vi "Unlock ECU Security.vi"(6 "Diagnostic Protocol":T2, 8 "error in (no error)":errorcluster, 10 "Security":T1={"Source DLL Path"=path "", "Security Level"=1, "Target DLL Path"=path ""}, 11 "diag ref in":T3) -> (0 "error out":errorcluster, 1 "success?":bool, 3 "diag ref out":T3)   [LabVIEW 2015, in "Diagnostics Addon Engine.lvlib"]
uses:
  Diagnostics Addon Engine.lvlib
  <vilib>/Automotive Diagnostic Command Set/Diagnostic Transport.llb/Diag Reference.ctl
  <vilib>/Automotive Diagnostic Command Set/Diagnostic Transport.llb/Transport Protocol Selector.ctl
  <vilib>/Automotive Diagnostic Command Set/Diagnostic Transport.llb/Diag CAN Frame Log.ctl
  Shared/Diagnostic Protocols.ctl
  Shared/Security.ctl
  GMLAN/_SubVIs/SecurityAccess_sendKey.vi
  GMLAN/_SubVIs/SecurityAccess_requestSeed.vi
  <vilib>/Automotive Diagnostic Command Set/Diagnostic Transport.llb/Apply Success Failure Error.vi
  <vilib>/Automotive Diagnostic Command Set/Diagnostic Transport.llb/Diagnostic Service.vi
  GMLAN/GMLAN.lvlib
  <vilib>/addons/Automotive Diagnostic Command Set/NI_Automotive Diagnostic Command Set.lvlib
  Shared/Diagnostics Addon Shared.lvlib
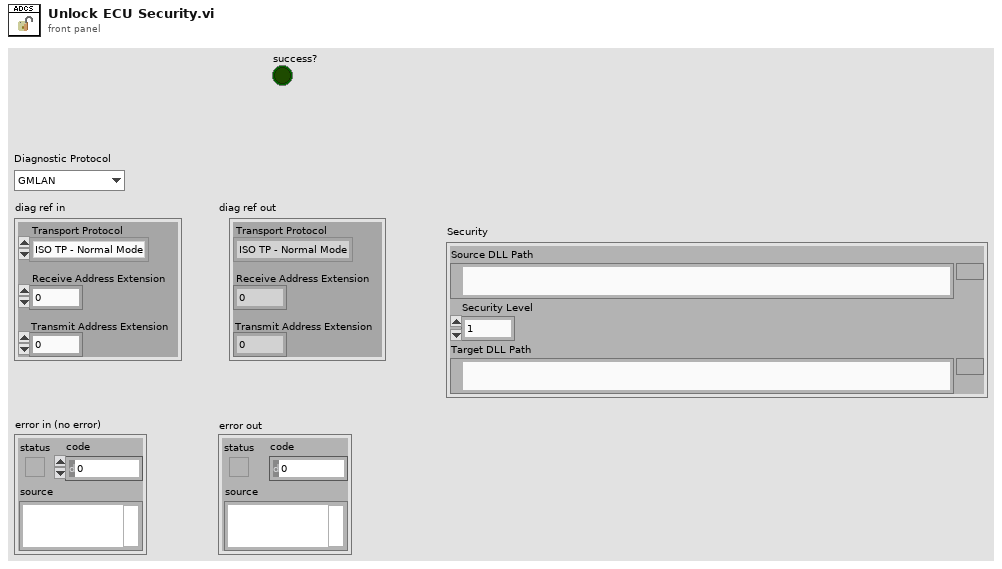
[diagram p1: front panel]
types:
  T1 = typedef "Diagnostics Addon Shared.lvlib/Security.ctl" = cluster{"Source DLL Path":path, "Security Level":u8, "Target DLL Path":path}
  T2 = typedef "Diagnostics Addon Shared.lvlib/Diagnostic Protocols.ctl" = enum16{"GMLAN", "KWP-2000", "UDS"}
  T3 = typedef "NI_Automotive Diagnostic Command Set.lvlib/Diag Reference.ctl" = cluster{"Diag CAN Handle":u32, "Transport Protocol":T4, "Receive Address Extension":u8, "Transmit Address Extension":u8, "Receive CAN Id":u32, "Transmit CAN Id":u32, "Diag CAN Queue":refnum<queue>, "Log Frames ?":bool, "My TP Address":u8, "Other TP Address":u8, "T1":u16, "T2":u16, "T3":u16, "T4":u16, "Tx SN":u8, "Block Size":u8, "Rx SN":u8, "VW TP Initialized?":bool, "Tx block no":u8, "baud rate":u32, "Interface":string, "Channel Diag CAN Handle":u32, "UDP Connection ID":refnum<k16>, "TCP Connection ID":refnum<k5>, "Target IP Addr":u32, "Source Address":u16, "Target Address":u16, "Send Header NACK?":bool, "DLL Handle":u32, "NAD":u8, "Time Stamp read first":dbl, "Time Stamp read last":dbl, "Time Stamp write first":dbl, "Time Stamp write last":dbl, "Time Stamp write":dbl, "Time Stamp read":dbl}
  T4 = typedef "NI_Automotive Diagnostic Command Set.lvlib/Transport Protocol Selector.ctl" = enum16{"ISO TP - Normal Mode", "ISO TP - Mixed Mode", "VW TP 2.0", "Diagnostics on IP", "ISO TP LIN"}
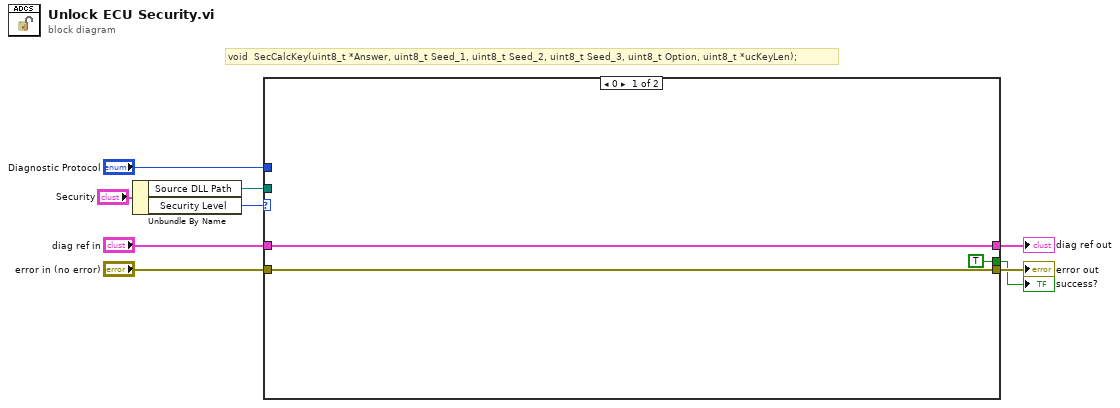
[diagram p0: block diagram]
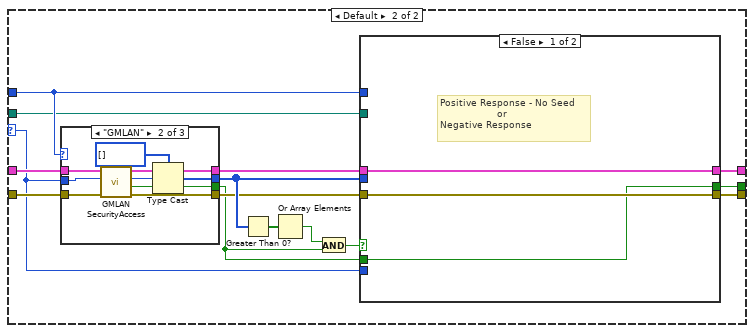
[diagram p2: hidden frame]
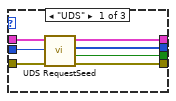
[diagram p3: hidden frame]
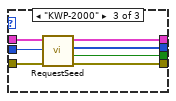
[diagram p4: hidden frame]
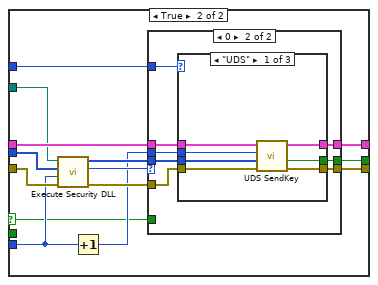
[diagram p5: hidden frame]
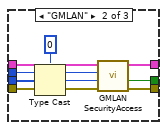
[diagram p7: hidden frame]
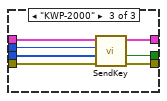
[diagram p8: hidden frame]
diagram:
  # "void  SecCalcKey(uint8_t *Answer, uint8_t Seed_1, uint8_t Seed_2, uint8_t Seed_3, uint8_t Option, uint8_t *ucKeyLen);"
  n1 = Unbundle By Name("Security") -> ("Source DLL Path"=w3:path, "Security Level"=w2:u8)
  n2 = case shown="0" w2 {
    selector: w2 -> [_ w15]
    tunnel: "diag ref in" -> [w12 w27]
    tunnel: [w12 w26] -> w8
    tunnel: "Diagnostic Protocol" -> [_ w22]
    tunnel: "error in (no error)" -> [w11 w19]
    tunnel: [w11 w17] -> w5
    tunnel: w3 -> [_ w16]
    tunnel: [TRUE ("success?") w13] -> w1
    frame 0 {
    }
    frame Default {
      n3 = case shown="\"GMLAN\"" w22 {
        tunnel: w19 -> [w31 w41 w50]
        tunnel: w27 -> [w32 w43 w49]
        tunnel: [w28 w38 w48] -> w21
        tunnel: w15 -> [w33 w42 w47]
        tunnel: [w30 w40 w46] -> w18
        tunnel: [w29 w35 w45] -> w20
        tunnel: [w34 w39 w44] -> w14
        frame "UDS" {
          n4 = call <vilib>:"UDS RequestSeed.vi"("error in (no error)"=w31, "access mode"=w33, "diag ref in"=w32) -> ("error out"=w30:errorcluster, "success?"=w34:bool, "seed out"=w29:u8[], "diag ref out"=w28:T3)  [unwired: 5 in]
        }
        frame "GMLAN" {
          n5 = call-poly "GMLAN SecurityAccess.vi"("error in (no error)"=w41, "subFunction"=w42, "diag ref in"=w43) -> ("error out"=w40:errorcluster, "success?"=w39:bool, "SecuritySeed"=w37:u16, "diag ref out"=w38:T3)  [unwired: 5 in]
          n6 = Type Cast(type=u8[] [] ("seed out"), x=w37) -> (*(type *) &x=w35:u8[])
        }
        frame "KWP-2000" {
          n7 = call <vilib>:"RequestSeed.vi"("error in (no error)"=w50, "access mode"=w47, "diag ref in"=w49) -> ("error out"=w46:errorcluster, "success?"=w44:bool, "seed out"=w45:u8[], "diag ref out"=w48:T3)  [unwired: 5 in]
        }
      }
      n8 = Greater Than 0?(x=w20) -> (x > 0?=w25:bool[])
      n9 = Or Array Elements(Boolean array=w25) -> (logical OR=w23:bool)
      n10 = And(x=w23, y=w14) -> (x .and. y?=w24:bool)
      n11 = case shown="False" w24 {
        selector: w24 -> [_ w55]
        tunnel: [w52 w67] -> w17
        tunnel: w16 -> [_ w61]
        tunnel: w21 -> [w53 w66]
        tunnel: w20 -> [_ w62]
        tunnel: w18 -> [w52 w63]
        tunnel: [w53 w65] -> w26
        tunnel: w15 -> [_ w57]
        tunnel: w22 -> [_ w64]
        tunnel: [w51 w54] -> w13
        tunnel: w14 -> [w51 _]
        frame False {
          # "Positive Response - No Seed\n                   or\nNegative Response"
        }
        frame True {
          n12 = call "Execute Security DLL.vi"("error in (no error)"=w63, "Option"=w57, "Seed"=w62, "path in"=w61) -> ("error out"=w58:errorcluster, "lockstatus"=w59:u8, "unsigned byte array"=w60:u8[])  [unwired: 5 in]
          n13 = Increment(x=w57) -> (x+1=w56:u8)
          n14 = case shown="0" w59 {
            tunnel: [w70 w78] -> w67
            tunnel: w66 -> [w69 w77]
            tunnel: [w69 w76] -> w65
            tunnel: w56 -> [_ w75]
            tunnel: w64 -> [_ w74]
            tunnel: w58 -> [w70 w73]
            tunnel: w60 -> [_ w72]
            tunnel: [w68 w71] -> w54
            tunnel: w55 -> [w68 _]
            frame Default {
            }
            frame 0 {
              n15 = case shown="\"UDS\"" w74 {
                tunnel: [w83 w91 w101] -> w78
                tunnel: w77 -> [w85 w93 w100]
                tunnel: w73 -> [w82 w92 w99]
                tunnel: [w84 w90 w98] -> w76
                tunnel: w75 -> [w80 w94 w97]
                tunnel: w72 -> [w81 w89 w96]
                tunnel: [w79 w86 w95] -> w71
                frame "UDS" {
                  n16 = call <vilib>:"UDS SendKey.vi"("error in (no error)"=w82, "key in"=w81, "access mode"=w80, "diag ref in"=w85) -> ("error out"=w83:errorcluster, "success?"=w79:bool, "diag ref out"=w84:T3)  [unwired: 5 in]
                }
                frame "GMLAN" {
                  n17 = Type Cast(type=u16 0 ("SecuritySeed"), x=w89) -> (*(type *) &x=w88:u16)
                  n18 = call-poly "GMLAN SecurityAccess.vi"("error in (no error)"=w92, "SecuritySeed"=w88, "subFunction"=w94, "diag ref in"=w93) -> ("error out"=w91:errorcluster, "success?"=w86:bool, "diag ref out"=w90:T3)  [unwired: 5 in]
                }
                frame "KWP-2000" {
                  n19 = call <vilib>:"SendKey.vi"("error in (no error)"=w99, "key in"=w96, "access mode"=w97, "diag ref in"=w100) -> ("error out"=w101:errorcluster, "success?"=w95:bool, "diag ref out"=w98:T3)  [unwired: 5 in]
                }
              }
            }
          }
        }
      }
    }
  }
  "error out" <- w5
  "diag ref out" <- w8
  "success?" <- w1
